vi "Table Paste Clipboard.vi"(1 "signaling change (False)":bool, 2 "table ref":refnum<vi>) -> (0 "output data":string[][](array[string]))   [LabVIEW 2020]
doc: "Pastes clipboard matrix to table control."
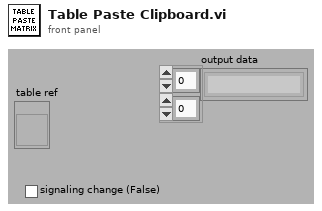
[diagram p1: front panel]
types:
  T1 = typedef "LVRowAndColumnTypeDef.ctl" = cluster{"Row":i32, "Column":i32}
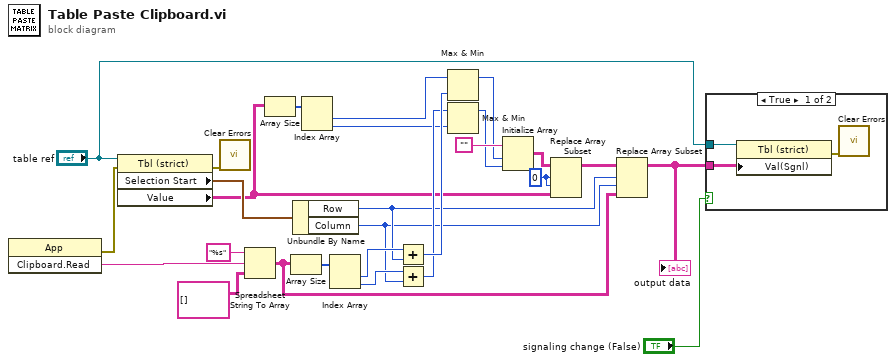
[diagram p0: block diagram]
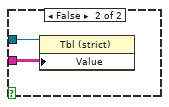
[diagram p2: hidden frame]
diagram:
  w5 = 0 ("index (row)")
  n1 = invoke class="App" method="Clipboard.Read"() -> (error out=w1:errorcluster, "Read Clipbrd"=w27:string)  [unwired: 3 in, 1 out]
  n2 = property on="Property Node" class="Tbl (strict)"(reference="table ref", error in=w1) -> (error out=w2:errorcluster, "Selection Start"=w24:T1, "Value"=w11:string[][])  [unwired: 1 out]
  n3 = call <vilib>:"Clear Errors.vi"("error in (no error)"=w2) -> ()  [unwired: 5 in, 2 out]
  n4 = Spreadsheet String To Array(format string="%s", spreadsheet string=w27, array type (2D Dbl)=string[][] []) -> (array=w7:string[][])  [unwired: 1 in]
  n5 = Array Size(array=w11) -> (size(s)=w23:i32[])
  n6 = Array Size(array=w7) -> (size(s)=w21:i32[])
  n7 = Unbundle By Name(w24) -> ("Row"=w9:i32, "Column"=w8:i32)
  n8 = Index Array(array=w23) -> (element #1=w13:i32, element #2=w12:i32)  [unwired: 2 in]
  n9 = Index Array(array=w21) -> (element #1=w20:i32, element #2=w19:i32)  [unwired: 2 in]
  n10 = Add(x=w20, y=w9) -> (x+y=w18:i32)
  n11 = Add(x=w19, y=w8) -> (x+y=w17:i32)
  n12 = Max & Min(x=w13, y=w18) -> (max(x,y)=w16:i32)  [unwired: 1 out]
  n13 = Max & Min(x=w17, y=w12) -> (max(x,y)=w15:i32)  [unwired: 1 out]
  n14 = Initialize Array("", w16, w15) -> (w14:string[][])
  n15 = Replace Array Subset(array=w14, new element=w11, index (row)=w5, index (col)=w5) -> (w10:string[][])
  n16 = Replace Array Subset(array=w10, new element=w7, index (row)=w9, index (col)=w8) -> (w6:string[][])
  "output data" <- w6
  n17 = case shown="True" "signaling change (False)" {
    tunnel: w6 -> [w30 w32]
    tunnel: "table ref" -> [w29 w31]
    frame True {
      n18 = property on="Property Node" class="Tbl (strict)"(reference=w29, "Val(Sgnl)"=w30) -> (error out=w28:errorcluster)  [unwired: 1 in, 1 out]
      n19 = call <vilib>:"Clear Errors.vi"("error in (no error)"=w28) -> ()  [unwired: 5 in, 2 out]
    }
    frame False {
      n20 = property on="Property Node" class="Tbl (strict)"(reference=w31, "Value"=w32) -> ()  [unwired: 1 in, 2 out]
    }
  }
